vi "Set Result Settings.vi"(8 "error in (no error)":errorcluster, 10 "Analyze Parameter":refnum<class "Analyze Results Base.lvclass">, 11 "Analyze Compound Analysis Base in":refnum<class "Analyze Compound Analysis Base.lvclass">) -> (0 "error out":errorcluster, 3 "Analyze Compound Analysis Base out":refnum<class "Analyze Compound Analysis Base.lvclass">)   [LabVIEW 2020, in "Analyze.lvlib" / "Analyze Compound Analysis Base.lvclass"]
uses:
  Analyze Compound Analysis Base.lvclass
  Results and Overlays/Results Base/Analyze Results Base.lvclass
  Analyze Compound Analysis Base.lvclass/Analyze Compound Analysis Base.ctl
  Results and Overlays/Compound Results/Analyze Compound Results Base.lvclass
  Analyze BaseClass/Analyze BaseClass/Analyze BaseClass.lvclass
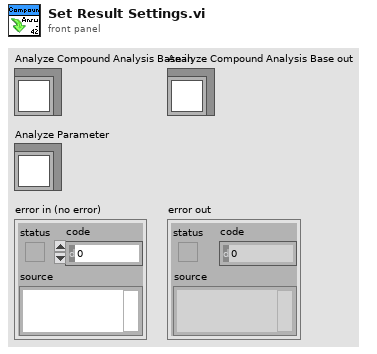
[diagram p1: front panel]
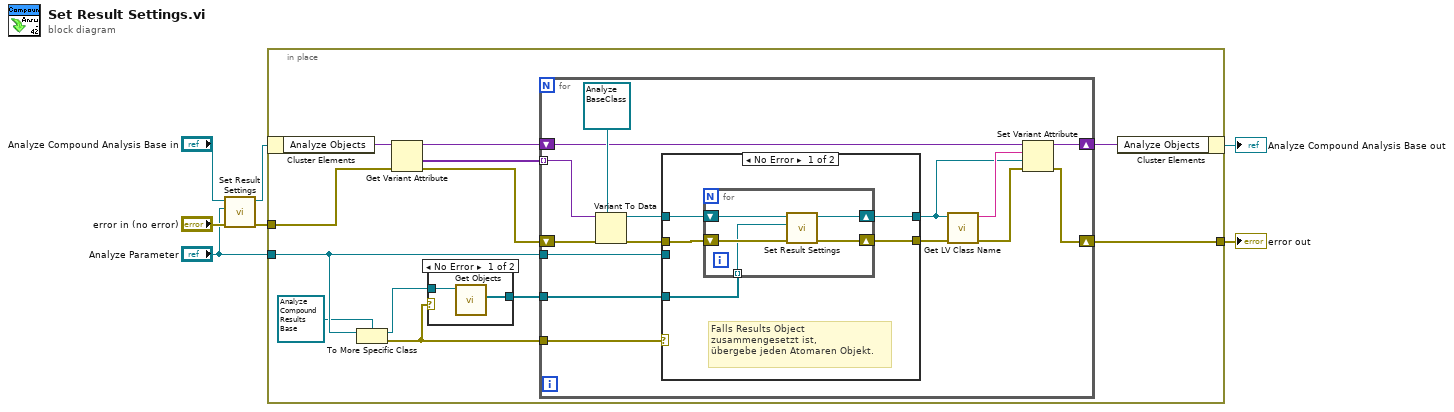
[diagram p0: block diagram]
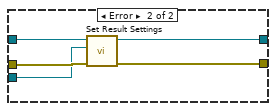
[diagram p3: hidden frame]
diagram:
  n1 = call-parent "Set Result Settings.vi"("error in (no error)"="error in (no error)", "Analyze Parameter"="Analyze Parameter", "Analyze BaseClass in"="Analyze Compound Analysis Base in") -> ("error out"=w4:errorcluster, "Analyze BaseClass out"=w3:refnum<class "Analyze Compound Analysis Base.lvclass">)  [unwired: 7 in]
  n2 = in-place {
    in-place-border: w4 -> [w14]
    in-place-border: [w17] -> w1
    in-place-border: "Analyze Parameter" -> [w12]
    n3 = in-place-cluster #1(w3) -> ("Analyze Objects"=w19:variant)
    n4 = To More Specific Class(target class=refnum<class "Analyze Compound Results Base.lvclass"> refnum ("Analyze Compound Results Base.lvclass"), reference=w12) -> (specific class reference=w9:refnum<class "Analyze Compound Results Base.lvclass">, error out=w10:errorcluster)  [unwired: 1 in]
    n5 = Get Variant Attribute(Variant=w19, error in=w14) -> (duplicate Variant=w16:variant, values=w18:variant[], error out=w13:errorcluster)  [unwired: 2 in, 1 out]
    n6 = case shown="No Error" w10 {
      tunnel: w9 -> [w21 _]
      tunnel: [w20 _] -> w8
      frame No Error {
        n7 = call "Get Objects.vi"("Analyze Compound Results Base in"=w21) -> ("Result Objs"=w20:refnum<class "Analyze Results Base.lvclass">[])  [unwired: 8 in, 2 out]
      }
      frame Error {
      }
    }
    n8 = for {
      tunnel: w18 -> [w35] mode=indexing
      shift-right: [w30] -> w17
      shift-left: w13 -> [w34]
      shift-right: [w32] -> w15
      shift-left: w16 -> [w33]
      tunnel: w12 -> [w26]
      tunnel: w10 -> [w23]
      tunnel: w8 -> [w22]
      n9 = Variant To Data(error in=w34, type=refnum<class "Analyze BaseClass.lvclass"> refnum ("Analyze.lvlib:Analyze BaseClass.lvlib:Analyze BaseClass.lvclass"), Variant=w35) -> (data=w28:refnum<class "Analyze BaseClass.lvclass">, error out=w27:errorcluster)
      n10 = case shown="No Error" w23 {
        tunnel: w28 -> [w41 w51]
        tunnel: w27 -> [w38 w50]
        tunnel: w26 -> [_ w49]
        tunnel: [w40 w48] -> w25
        tunnel: [w39 w47] -> w24
        tunnel: w22 -> [w37 _]
        frame No Error {
          # "Falls Results Object \nzusammengesetzt ist,\nübergebe jeden Atomaren Objekt."
          n11 = for {
            shift-right: [w45] -> w40
            shift-left: w41 -> [w46]
            shift-right: [w44] -> w39
            shift-left: w38 -> [w43]
            tunnel: w37 -> [w42] mode=indexing
            n12 = call-dynamic "Set Result Settings.vi"("error in (no error)"=w43, "Analyze Parameter"=w42, "Analyze BaseClass in"=w46) -> ("error out"=w44:errorcluster, "Analyze BaseClass out"=w45:refnum<class "Analyze BaseClass.lvclass">)  [unwired: 7 in]
          }
        }
        frame Error {
          n13 = call-dynamic "Set Result Settings.vi"("error in (no error)"=w50, "Analyze Parameter"=w49, "Analyze BaseClass in"=w51) -> ("error out"=w47:errorcluster, "Analyze BaseClass out"=w48:refnum<class "Analyze BaseClass.lvclass">)  [unwired: 7 in]
        }
      }
      n14 = call <vilib>:"Get LV Class Name.vi"("error in (no error)"=w24, "object"=w25) -> ("error out"=w31:errorcluster, "class name"=w29:string)  [unwired: 8 in]
      n15 = Set Variant Attribute(Variant=w33, name=w29, value=w25, error in=w31) -> (Variant out=w32:variant, error out=w30:errorcluster)  [unwired: 1 out]
    }
    n16 = in-place-cluster #1("Analyze Objects"=w15) -> (→"Analyze Compound Analysis Base out":refnum<class "Analyze Compound Analysis Base.lvclass">)
  }
  "error out" <- w1
